vi "io_query_long_data.vi"(4 "Simulation read buffer (\"Simulation\")":string="Simulation", 8 "error in":errorcluster caption="error in (no error)", 10 "write buffer":string, 11 "VISA resource name":refnum<visa-resource-name>) -> (0 "error out":errorcluster, 2 "read buffer":string, 3 "VISA resource name out":refnum<visa-resource-name>)   [LabVIEW 2022 SP3, in "hmp4000_rsidr_core.lvlib"]
uses:
  hmp4000_rsidr_core.lvlib
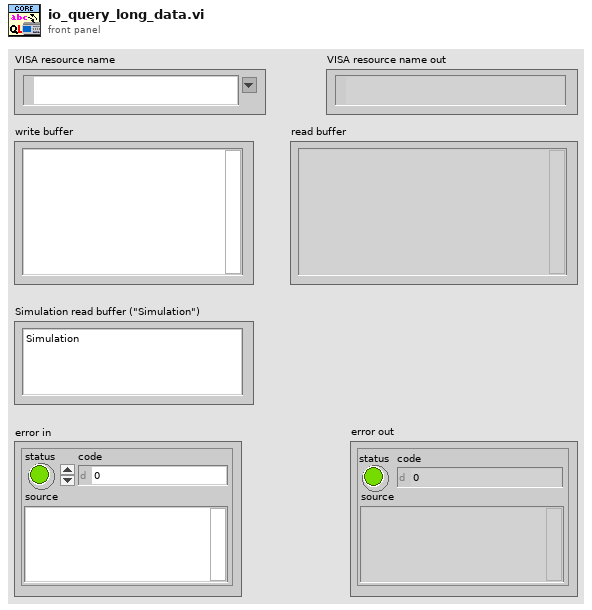
[diagram p1: front panel]
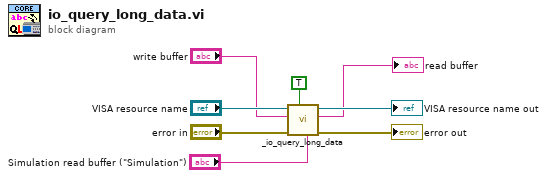
[diagram p0: block diagram]
diagram:
  n1 = call "_io_query_long_data.vi"("Simulation read buffer (\"Simulation\")"="Simulation read buffer (\"Simulation\")", "Trim Response End"=TRUE ("Trim Response End (T)"), "error in"="error in", "Write buffer"="write buffer", "VISA resource name"="VISA resource name") -> ("error out"=→"error out":errorcluster, "Read buffer"=→"read buffer":string, "VISA resource name out"=→"VISA resource name out":refnum<visa-resource-name>)  [unwired: 4 in]
